vi "myRIO Customized FPGA.vi"() -> ()   [LabVIEW 2019]
uses:
  <vilib>/Platform/TimedLoop/XDataNode/timing_clust.ctl
  <vilib>/Platform/TimedLoop/XDataNode/nitl_modes.ctl
  <vilib>/Platform/TimedLoop/XDataNode/wakeup.ctl
  <vilib>/rvi/Emulation/niFpgaSctlEmulationGetInTimedLoop.vi
  <vilib>/rvi/Emulation/niFpgaEmulationReportErrorSimple.vi
  <vilib>/rvi/Emulation/niFpgaGetClockAttributes.vi
  <vilib>/rvi/Emulation/niFpgaCriticalErrorInLSC.vi
  <vilib>/rvi/eio/common/nirviEmuTemplateMethod_errors.vi
  <vilib>/rvi/interface/RandomDataEmulation/niFpgaRandomDataHandleErrors.vi
  <vilib>/rvi/Emulation/niFpgaProcessEmulError.vi
  <vilib>/Platform/TimedLoop/XDataNode/XDataNode.xnode
  <vilib>/eio/EIONode/EIONode.xnode
  <vilib>/rvi/DataTransferAndStorage/Container/XNode/niFpgaContainer.xnode
  <vilib>/rvi/interface/RandomDataEmulation/nirviRandomDataFpgaReadWriteTemplate.vi
  <vilib>/Platform/TimedLoop/XDataNode/XDNodeRunTimeDep.lvlib
panel:
  out "24V Error":bool
  in  "myRIO LED3:0":u8
  out "myRIO Button":u8
  out "Stall Warning 0":bool
  out "Stall Error 1":bool
  out "Stall Warning 1":bool
  out "Stall Error 0":bool
  in  "LED2 Red":bool
  in  "LED3 Red":bool
  in  "LED3 Yellow":bool
  in  "LED3 Green":bool
  in  "LED2 Yellow":bool
  in  "LED2 Green":bool
  in  "LED1 Red":bool
  in  "LED1 Yellow":bool
  in  "LED1 Green":bool
  in  "Calibrated":bool
  out "FIFO Receive Time Out":bool
  out "Framing Error":bool
  in  "Clear Framing Error":bool
  in  "UART Clock Divisor":u16
  in  "Camera Power":bool
  in  "PWM.1A":u16
  in  "PWM.1B":u16
  in  "PWM1 Enable":bool
  out "Encoder 1 Raw":fxp<+,2,2> format="%02b"
  in  "PWM.0A":u16
  in  "PWM.0B":u16
  out "Encoder 0 Raw":fxp<+,2,2> format="%02b"
  in  "PWM0 Enable":bool
  in  "Encoder 0 Reset":bool
  in  "Encoder 1 Reset":bool
  out "Encoder 1 Counter":i32
  out "Encoder 0 Counter":i32
  in  "Encoder 0 Reset Value":i32
  in  "Encoder 1 Reset Value":i32
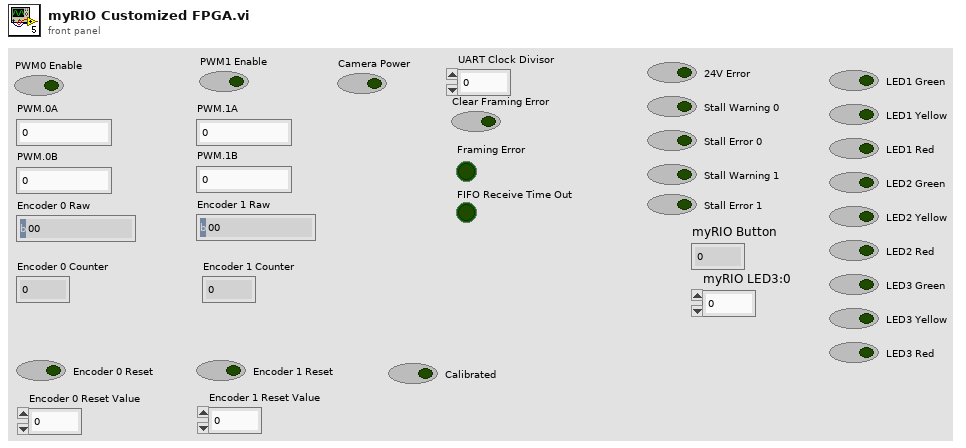
[diagram p1: front panel]
types:
  T1 = enum16{"Idle", "Testing Start", "Finish Start", "Data", "FIFO Data", "Testing Stop"}
  T2 = enum16{"Idle", "Send Bit", "Wait for Baud Period"}
  T3 = typedef "XDNodeRunTimeDep.lvlib/timing_clust.ctl" = cluster{"Expected End [f-1]":u64, "Actual End [f-1]":u64, "Finished Late? [f-1]":bool, "Expected End [i-1]":u64, "Actual End [i-1]":u64, "Finished Late? [i-1]":bool, "Expected Start [i]":u64, "Actual Start [i]":u64, "Expected Start [f]":u64, "Actual Start [f]":u64, "Source Name":string, "Structure Name":string, "Period":i64, "Deadline":i64, "Offset":i64, "Start":i64, "Priority":i32, "Timeout":i32, "Mode":T4, "Wakeup Reason":T5, "Error":errorcluster, "Source Type":string, "Secondary Source Type":string, "Global End Time":u64, "Global Start Time":u64, "Frame Duration":u64, "Iteration Duration":u64, "Assigned CPU":i32, "I/O Scan Engine Mode":u32}
  T4 = typedef "XDNodeRunTimeDep.lvlib/nitl_modes.ctl" = enum32{"No Change", "Process missed periods, maintain original phase", "Discard missed periods, maintain original phase", "Process missed periods, ignore original phase", "Discard missed periods, ignore original phase"}
  T5 = typedef "XDNodeRunTimeDep.lvlib/wakeup.ctl" = enum32{"Normal", "Aborted", "Asynchronous wakeup", "Timing source error", "Timed loop error", "Timeout"}
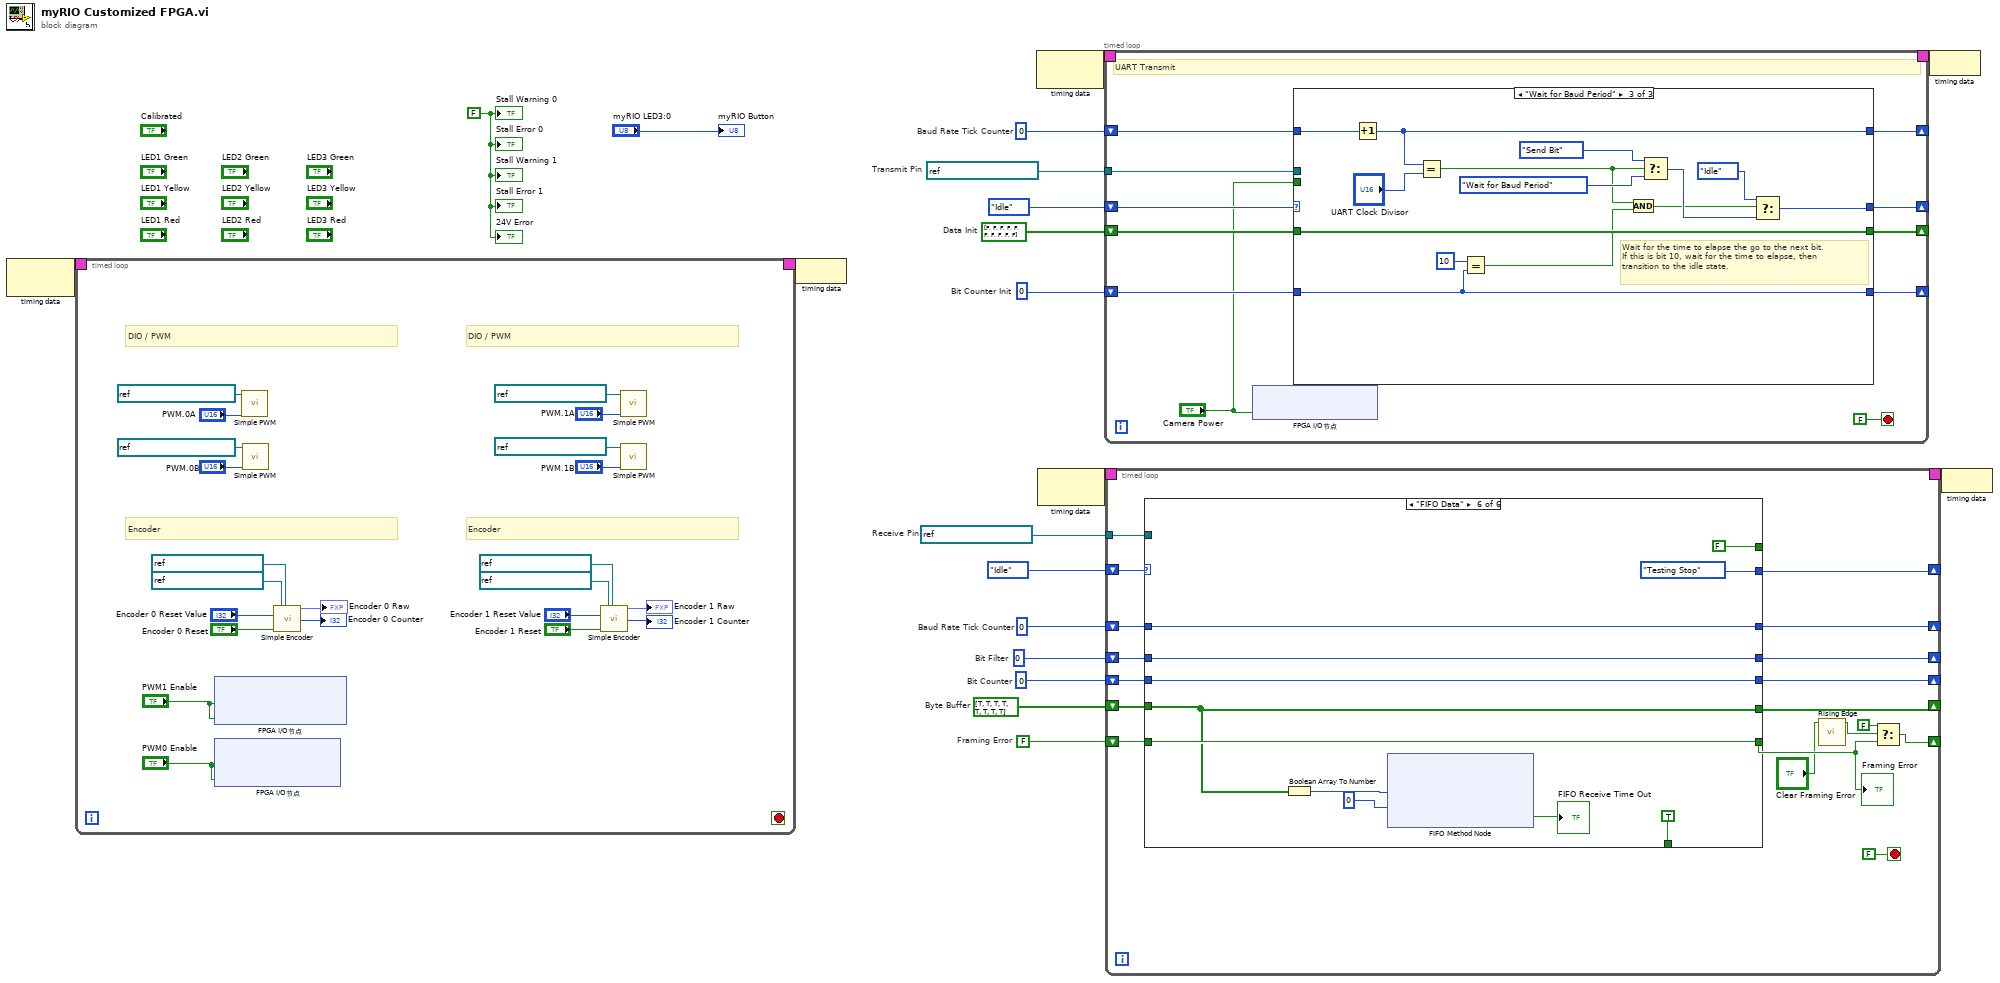
[diagram p0: block diagram]
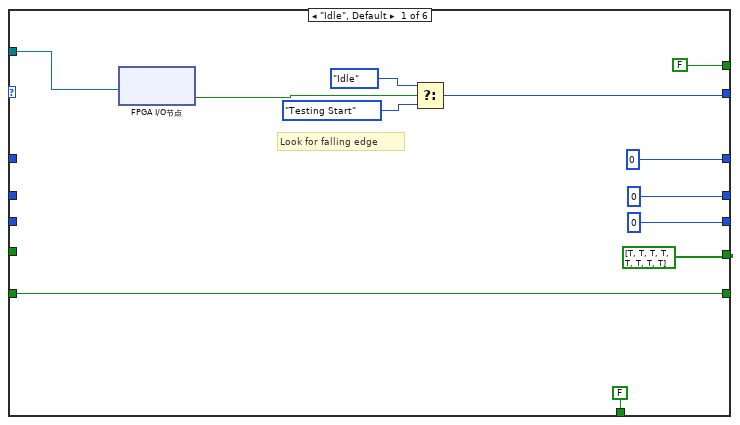
[diagram p2: hidden frame]
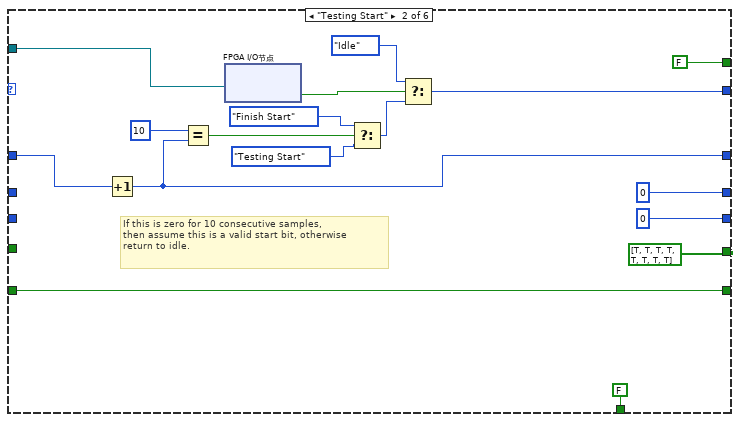
[diagram p3: hidden frame]
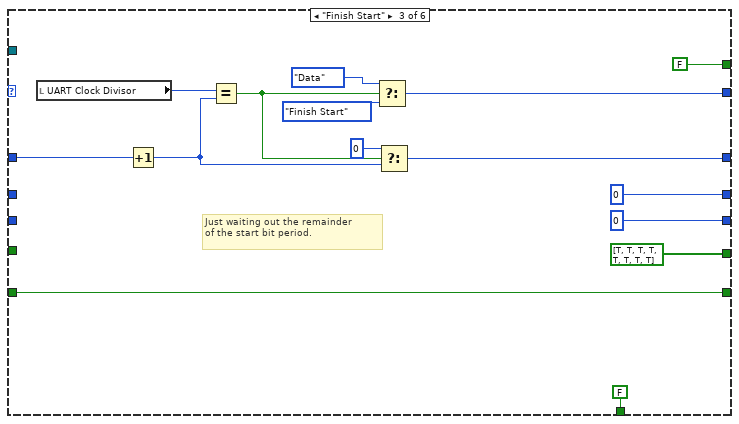
[diagram p4: hidden frame]
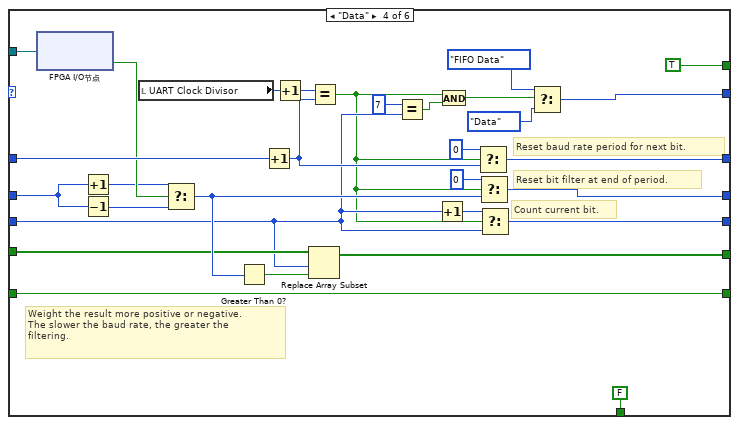
[diagram p5: hidden frame]
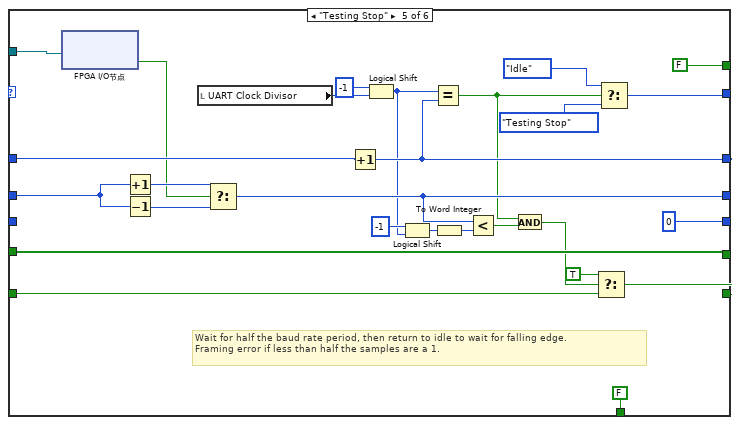
[diagram p6: hidden frame]
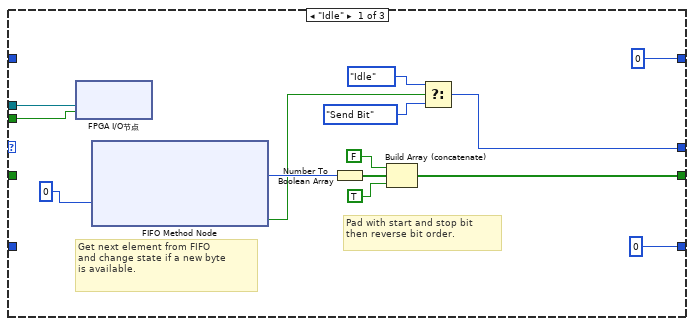
[diagram p7: hidden frame]
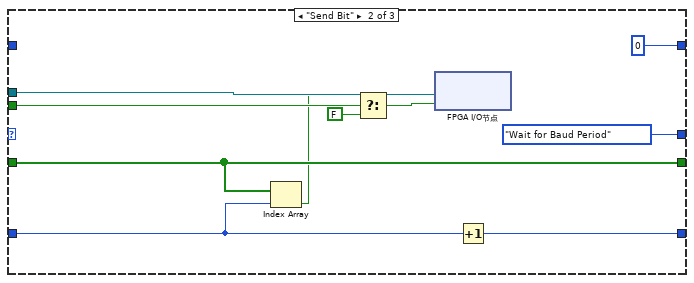
[diagram p8: hidden frame]
diagram:
  w1 = FALSE ("LED3 Green 6")
  w3 = bool[] [TRUE, TRUE, TRUE, TRUE, TRUE, TRUE, TRUE, TRUE]  # Byte Buffer
  w4 = i16 0  # Bit Filter
  w5 = FALSE  # Framing Error
  w6 = u16 0  # Bit Counter
  w7 = u16 0  # Baud Rate Tick Counter
  w9 = refnum<k21> "ConnectorC/DIO2"  # Transmit Pin
  w8 = refnum<k21> "ConnectorB/DIO2"  # Receive Pin
  w11 = bool[] [FALSE, FALSE, FALSE, FALSE, FALSE, FALSE, FALSE, FALSE, FALSE, FALSE]  # Data Init
  w12 = 0  # Bit Counter Init
  w14 = u16 0  # Baud Rate Tick Counter
  n1 = node-c288() -> (w20:T3)  [unwired: 1 in]
  n2 = timed-loop {
    timing: w20 -> [_]
    timing-out: [_] -> w19
    stop <- _ stop-if-true
    # "Encoder"
    # "DIO / PWM"
    # "Encoder"
    # "DIO / PWM"
    n3 = xnode "FPGA I/O节点"("ConnectorA/DIO6"="PWM1 Enable", "ConnectorA/DIO12"="PWM1 Enable") -> ()  [unwired: 2 in, 2 out]
    n4 = xnode "FPGA I/O节点"("ConnectorA/DIO9"="PWM0 Enable", "ConnectorA/DIO2"="PWM0 Enable") -> ()  [unwired: 2 in, 2 out]
    n5 = call "Simple PWM.vi"("Compare Value"="PWM.0A", "PWM"=refnum<k21> "ConnectorA/DIO11" ("DIO/PWM")) -> ()  [unwired: 10 in]
    n6 = call "Simple PWM.vi"("Compare Value"="PWM.0B", "PWM"=refnum<k21> "ConnectorA/DIO10" ("DIO/PWM")) -> ()  [unwired: 10 in]
    n7 = call "Simple Encoder.vi"("Encoder Reset Value"="Encoder 0 Reset Value", "Encoder Reset"="Encoder 0 Reset", "DIO.1/QE.B"=refnum<k21> "ConnectorC/DIO4", "DIO.0/QE.A"=refnum<k21> "ConnectorC/DIO6") -> ("RAW A/B"=→"Encoder 0 Raw":fxp<+,2,2>, "Counter"=→"Encoder 0 Counter":i32)  [unwired: 14 in]
    n8 = call "Simple Encoder.vi"("Encoder Reset Value"="Encoder 1 Reset Value", "Encoder Reset"="Encoder 1 Reset", "DIO.1/QE.B"=refnum<k21> "ConnectorA/DIO0", "DIO.0/QE.A"=refnum<k21> "ConnectorA/DIO1") -> ("RAW A/B"=→"Encoder 1 Raw":fxp<+,2,2>, "Counter"=→"Encoder 1 Counter":i32)  [unwired: 14 in]
    n9 = call "Simple PWM.vi"("Compare Value"="PWM.1A", "PWM"=refnum<k21> "ConnectorA/DIO8" ("DIO/PWM")) -> ()  [unwired: 10 in]
    n10 = call "Simple PWM.vi"("Compare Value"="PWM.1B", "PWM"=refnum<k21> "ConnectorA/DIO4" ("DIO/PWM")) -> ()  [unwired: 10 in]
  }
  n11 = node-c288(w19) -> ()
  n12 = node-c288() -> (w18:T3)  [unwired: 1 in]
  n13 = node-c288() -> (w16:T3)  [unwired: 1 in]
  n14 = timed-loop {
    timing: w18 -> [_]
    timing-out: [_] -> w17
    shift-right: [w50] -> _
    shift-left: w14 -> [w51]
    shift-right: [w54] -> _
    shift-left: T2."Idle" -> [w55]
    shift-right: [w52] -> _
    shift-left: w12 -> [w53]
    shift-right: [w49] -> _
    shift-left: w11 -> [w48]
    tunnel: w9 -> [w46]
    stop <- FALSE stop-if-true
    # "UART Transmit"
    n15 = xnode "FPGA I/O节点"("ConnectorB/DIO3"="Camera Power") -> ()  [unwired: 1 in, 1 out]
    n16 = case shown="\"Wait for Baud Period\"" w55 {
      tunnel: [w69 T2."Wait for Baud Period" w87] -> w54
      tunnel: w53 -> [_ w79 w86]
      tunnel: [0 w78 w86] -> w52
      tunnel: w51 -> [_ _ w93]
      tunnel: [u16 0 u16 0 w92] -> w50
      tunnel: w48 -> [_ w75 w85]
      tunnel: [w61 w75 w85] -> w49
      tunnel: w46 -> [w60 w74 _]
      tunnel: "Camera Power" -> [w59 w73 _]
      frame "Idle" {
        # "Get next element from FIFO\nand change state if a new byte\nis available."
        # "Pad with start and stop bit\nthen reverse bit order."
        n17 = xnode "FPGA I/O节点"("I/O项"=w59, "FPGA I/O输入"=w60) -> ()  [unwired: 1 out]
        n18 = xnode ("FIFO Method Node")("超时"=0 ("Timeout")) -> ("元素"=w57:u8, "超时？"=w56:bool)  [unwired: 1 in, 1 out]
        n19 = Number To Boolean Array(number=w57) -> (Boolean array=w66:bool[])
        n20 = Build Array (concatenate)(FALSE, w66, TRUE) -> (w61:bool[])
        n21 = Select(t=T2."Idle", s=w56, f=T2."Send Bit") -> (s? t:f=w69:T2)
      }
      frame "Send Bit" {
        n22 = Index Array(array=w75, index=w79) -> (element=w72:bool)
        n23 = Select(t=w72, s=w73, f=FALSE) -> (s? t:f=w71:bool)
        n24 = xnode "FPGA I/O节点"("I/O项"=w71, "FPGA I/O输入"=w74) -> ()  [unwired: 1 out]
        n25 = Increment(x=w79) -> (x+1=w78:i32)
      }
      frame "Wait for Baud Period" {
        # "Wait for the time to elapse the go to the next bit.\nIf this is bit 10, wait for the time to elapse, then \ntransition to the idle state."
        n26 = Increment(x=w93) -> (x+1=w92:u16)
        n27 = Equal?(x=w92, y="UART Clock Divisor") -> (x = y?=w81:bool)
        n28 = Equal?(x=10, y=w86) -> (x = y?=w82:bool)
        n29 = And(x=w81, y=w82) -> (x .and. y?=w80:bool)
        n30 = Select(t=T2."Send Bit", s=w81, f=T2."Wait for Baud Period") -> (s? t:f=w83:T2)
        n31 = Select(t=T2."Idle", s=w80, f=w83) -> (s? t:f=w87:T2)
      }
    }
  }
  n32 = timed-loop {
    timing: w16 -> [_]
    timing-out: [_] -> w15
    shift-right: [w99] -> _
    shift-left: T1."Idle" -> [w100]
    tunnel: w8 -> [w112]
    shift-right: [w110] -> _
    shift-left: w7 -> [w111]
    shift-right: [w109] -> _
    shift-left: w6 -> [w105]
    shift-right: [w107] -> _
    shift-left: w5 -> [w108]
    shift-right: [w103] -> _
    shift-left: w4 -> [w104]
    shift-right: [w101] -> _
    shift-left: w3 -> [w102]
    stop <- FALSE stop-if-true
    n33 = case shown="\"FIFO Data\"" w100 {
      tunnel: [w124 w140 w156 w183 w209 T1."Testing Stop"] -> w99
      tunnel: w112 -> [w123 w142 _ w175 w205 _]
      tunnel: w111 -> [_ w139 w157 w184 w214 w225]
      tunnel: [u16 0 ("Baud Rate Tick Counter") w135 w150 w182 w210 w225] -> w110
      tunnel: [u16 0 ("Baud Rate Tick Counter") u16 0 ("Baud Rate Tick Counter") u16 0 ("Baud Rate Tick Counter") w180 u16 0 ("Bit Counter") w223] -> w109
      tunnel: [w120 w133 w149 w176 w190 w222] -> w98
      tunnel: w108 -> [w120 w133 w149 w176 w192 w222]
      tunnel: w105 -> [_ _ _ w166 _ w223]
      tunnel: w104 -> [_ _ _ w173 w202 w224]
      tunnel: [i16 0 ("Bit Filter") i16 0 ("Bit Filter") i16 0 ("Bit Filter") w169 w200 w224] -> w103
      tunnel: w102 -> [_ _ _ w167 w206 w220]
      tunnel: [bool[] [TRUE, TRUE, TRUE, TRUE, TRUE, TRUE, TRUE, TRUE] ("Byte Buffer") bool[] [TRUE, TRUE, TRUE, TRUE, TRUE, TRUE, TRUE, TRUE] ("Byte Buffer") bool[] [TRUE, TRUE, TRUE, TRUE, TRUE, TRUE, TRUE, TRUE] ("Byte Buffer") w164 w206 w220] -> w101
      tunnel: [FALSE FALSE FALSE TRUE FALSE FALSE] -> _
      tunnel: [FALSE FALSE FALSE FALSE FALSE TRUE] -> _
      frame "Idle", Default {
        # "Look for falling edge"
        n34 = xnode "FPGA I/O节点"("FPGA I/O输入"=w123) -> ("I/O项"=w125:bool)  [unwired: 1 out]
        n35 = Select(t=T1."Idle", s=w125, f=T1."Testing Start") -> (s? t:f=w124:T1)
      }
      frame "Testing Start" {
        # "If this is zero for 10 consecutive samples,\nthen assume this is a valid start bit, otherwise\nreturn to idle."
        n36 = Increment(x=w139) -> (x+1=w135:u16)
        n37 = Equal?(x=u16 10, y=w135) -> (x = y?=w137:bool)
        n38 = xnode "FPGA I/O节点"("FPGA I/O输入"=w142) -> ("I/O项"=w141:bool)  [unwired: 1 out]
        n39 = Select(t=T1."Finish Start", s=w137, f=T1."Testing Start") -> (s? t:f=w138:T1)
        n40 = Select(t=T1."Idle", s=w141, f=w138) -> (s? t:f=w140:T1)
      }
      frame "Finish Start" {
        # "Just waiting out the remainder\nof the start bit period."
        n41 = local read "UART Clock Divisor"() -> (w155:u16)
        n42 = Increment(x=w157) -> (x+1=w153:u16)
        n43 = Equal?(x=w155, y=w153) -> (x = y?=w151:bool)
        n44 = Select(t=T1."Data", s=w151, f=T1."Finish Start") -> (s? t:f=w156:T1)
        n45 = Select(t=u16 0, s=w151, f=w153) -> (s? t:f=w150:u16)
      }
      frame "Data" {
        # "Count current bit."
        # "Reset bit filter at end of period."
        # "Reset baud rate period for next bit."
        # "Weight the result more positive or negative.\nThe slower the baud rate, the greater the\nfiltering."
        n46 = xnode "FPGA I/O节点"("FPGA I/O输入"=w175) -> ("I/O项"=w174:bool)  [unwired: 1 out]
        n47 = Increment(x=w173) -> (x+1=w171:i16)
        n48 = Decrement(x=w173) -> (x-1=w172:i16)
        n49 = local read "UART Clock Divisor"() -> (w185:u16)
        n50 = Select(t=w171, s=w174, f=w172) -> (s? t:f=w168:i16)
        n51 = Greater Than 0?(x=w168) -> (x > 0?=w165:bool)
        n52 = Increment(x=w184) -> (x+1=w186:u16)
        n53 = Increment(x=w185) -> (x+1=w160:u16)
        n54 = Replace Array Subset(array=w167, new element=w165, index=w166) -> (w164:bool[])
        n55 = Equal?(x=w160, y=w186) -> (x = y?=w161:bool)
        n56 = Equal?(x=u16 7, y=w166) -> (x = y?=w178:bool)
        n57 = Increment(x=w166) -> (x+1=w179:u16)
        n58 = And(x=w161, y=w178) -> (x .and. y?=w181:bool)
        n59 = Select(t=u16 0, s=w161, f=w186) -> (s? t:f=w182:u16)
        n60 = Select(t=i16 0, s=w161, f=w168) -> (s? t:f=w169:i16)
        n61 = Select(t=w179, s=w161, f=w166) -> (s? t:f=w180:u16)
        n62 = Select(t=T1."FIFO Data", s=w181, f=T1."Data") -> (s? t:f=w183:T1)
      }
      frame "Testing Stop" {
        # "Wait for half the baud rate period, then return to idle to wait for falling edge.\nFraming error if less than half the samples are a 1."
        n63 = xnode "FPGA I/O节点"("FPGA I/O输入"=w205) -> ("I/O项"=w201:bool)  [unwired: 1 out]
        n64 = Increment(x=w202) -> (x+1=w203:i16)
        n65 = Decrement(x=w202) -> (x-1=w204:i16)
        n66 = local read "UART Clock Divisor"() -> (w212:u16)
        n67 = Select(t=w203, s=w201, f=w204) -> (s? t:f=w200:i16)
        n68 = Increment(x=w214) -> (x+1=w210:u16)
        n69 = Logical Shift(y=i16 -1, x=w212) -> (x << y=w197:u16)
        n70 = Logical Shift(y=i16 -1, x=w197) -> (x << y=w198:u16)
        n71 = Equal?(x=w197, y=w210) -> (x = y?=w194:bool)
        n72 = To Word Integer(number=w198) -> (16bit integer=w196:i16)
        n73 = Less?(x=w200, y=w196) -> (x < y?=w195:bool)
        n74 = And(x=w194, y=w195) -> (x .and. y?=w193:bool)
        n75 = Select(t=TRUE, s=w193, f=w192) -> (s? t:f=w190:bool)
        n76 = Select(t=T1."Idle", s=w194, f=T1."Testing Stop") -> (s? t:f=w209:T1)
      }
      frame "FIFO Data" {
        n77 = Boolean Array To Number(Boolean array=w220) -> (number=w217:u8)
        n78 = xnode ("FIFO Method Node")("元素"=w217, "超时"=0 ("Timeout")) -> ("超时？"=→"FIFO Receive Time Out":bool)  [unwired: 1 in, 1 out]
      }
    }
    "Framing Error" <- w98
    n79 = call "Rising Edge.vi"("Input"="Clear Framing Error") -> ("Rise?"=w96:bool)  [unwired: 10 in]
    n80 = Select(t=FALSE, s=w96, f=w98) -> (s? t:f=w107:bool)
  }
  n81 = node-c288(w17) -> ()
  n82 = node-c288(w15) -> ()
  "Stall Error 0" <- w1
  "Stall Warning 1" <- w1
  "Stall Error 1" <- w1
  "Stall Warning 0" <- w1
  "myRIO Button" <- "myRIO LED3:0"
  "24V Error" <- w1
